vi "模拟控件转String.vi"(1 "Input":T2={"Digital Start Trigger Source 4"="/Dev1/PFI0", "Digital Start Trigger Edge 4"=10280, "min volt (V)"=0.0, "max volt (V)"=1.0, "rate"=100000.0, "device name"="Dev1", "Formula In"=[], "Total time (s)"=0.0} {"rate" format="%0.2f"; "max volt (V)" format="%0.2f"; "min volt (V)" format="%0.2f"; "Digital Start Trigger Edge 4" items=["Rising"=10280, "Falling"=10171]}) -> (0 "output":T1={"Digital Start Trigger Source 4"="/Dev1/PFI0", "Digital Start Trigger Edge 4"="", "minimum value"=-10.0, "maximum value"=10.0, "rate"=1000.0, "device name"="PXI1Slot5", "Total time"=0.0, "Formula In"=[]} {"rate" format="%0.2f"; "maximum value" format="%0.2f"; "minimum value" format="%0.2f"})   [LabVIEW 2021]
panel:
  # "1、formular in 中sample为各个分段函数的持续时间。\n2、Total time 为总时间，必须大于sample加起来的值。\n3、minimum value和maximum value默认±10V不改。\n4、rate为采样率，即时钟频率\n5、device name为选择的板卡名字，可选为PXI1Slot5-7\n6、Source 为接受触发的端口，Edge为选择上升沿触发\n还是其他类型触发。"
  # "In0：780 VCO 幅值（初始 0.6）\nIn1：780 VCO 频率（初始 0.7）"
  # "1、Formula In 中 sample 为各个函数的持续时间\n2、Total time 为总时间，必须大于 sample 之和\n3、min volt 和 max volt 默认±10V\n4、rate 为采样率，即时钟频率\n5、device name 为选择的板卡，可选为 Dev1\n6、Source 为接受触发的端口，Edge 为触发类型"
  # "In0：780 VCO 幅值（初始 0.6）\nIn1：780 VCO 频率（初始 0.7）"
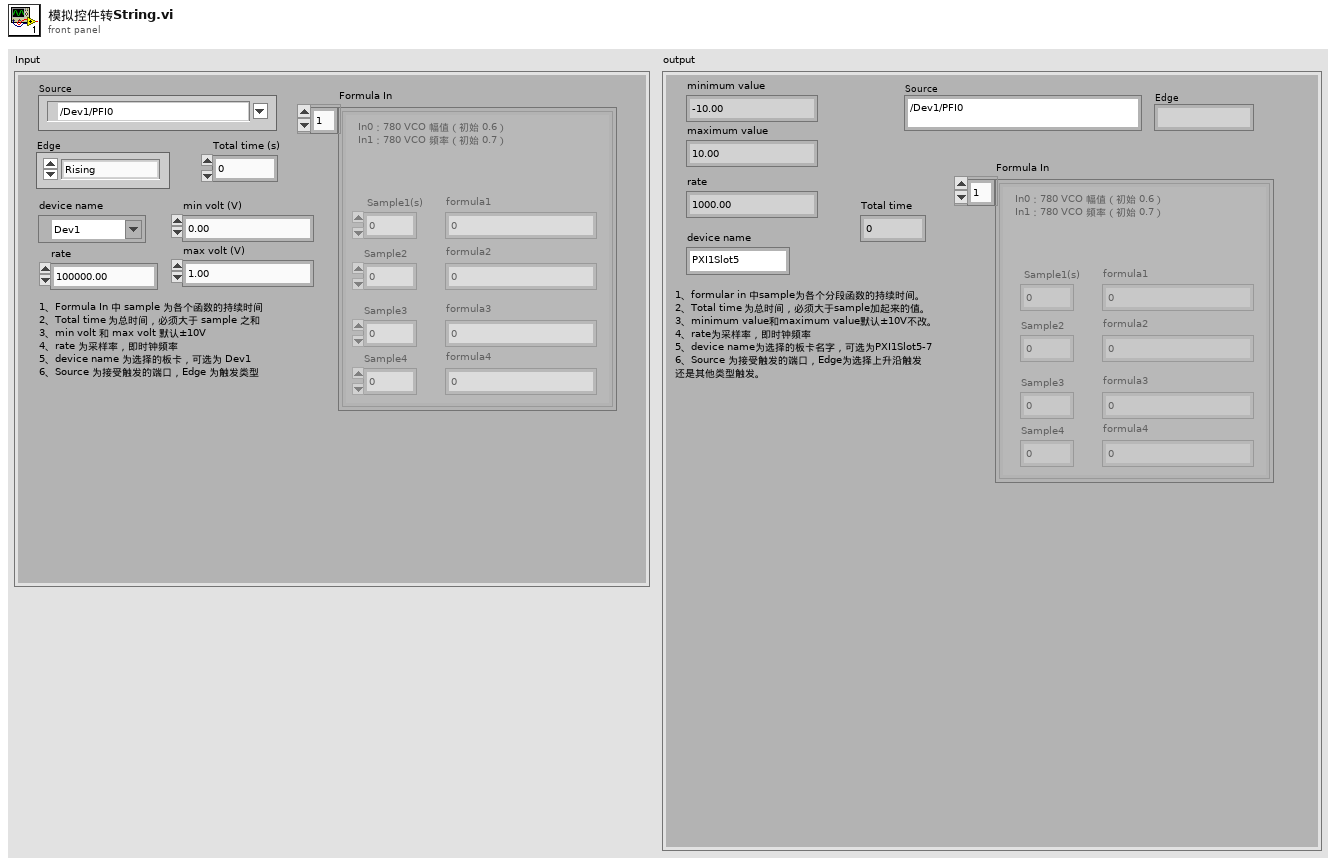
[diagram p1: front panel]
types:
  T1 = cluster{"Digital Start Trigger Source 4":string, "Digital Start Trigger Edge 4":string, "minimum value":dbl, "maximum value":dbl, "rate":dbl, "device name":string, "Total time":dbl, "Formula In":cluster{" Sample1(s)":dbl, "formula1":string, "Sample2":dbl, "formula2":string, "Sample3":dbl, "formula3":string, "Sample4":dbl, "formula4":string}[]}
  T2 = cluster{"Digital Start Trigger Source 4":tag, "Digital Start Trigger Edge 4":i32, "min volt (V)":dbl, "max volt (V)":dbl, "rate":dbl, "device name":tag, "Formula In":cluster{" Sample1(s)":dbl, "formula1":string, "Sample2":dbl, "formula2":string, "Sample3":dbl, "formula3":string, "Sample4":dbl, "formula4":string}[], "Total time (s)":dbl}
  T3 = cluster{" Sample1(s)":dbl, "formula1":string, "Sample2":dbl, "formula2":string, "Sample3":dbl, "formula3":string, "Sample4":dbl, "formula4":string}[]
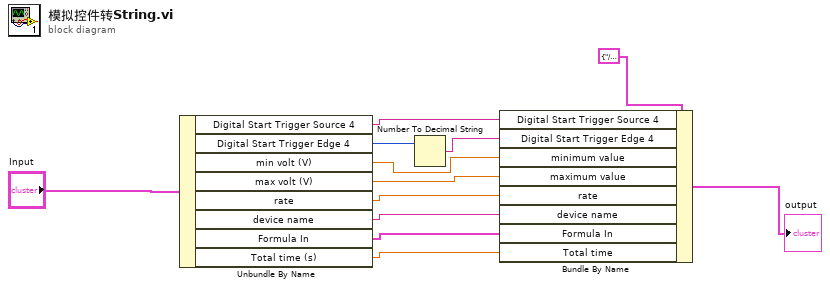
[diagram p0: block diagram]
diagram:
  n1 = Unbundle By Name("Input") -> ("Digital Start Trigger Source 4"=w9:tag, "Digital Start Trigger Edge 4"=w11:i32, "min volt (V)"=w7:dbl, "max volt (V)"=w6:dbl, "rate"=w5:dbl, "device name"=w4:tag, "Formula In"=w3:T3, "Total time (s)"=w2:dbl)
  n2 = Number To Decimal String(number=w11) -> (decimal integer string=w8:string)  [unwired: 1 in]
  n3 = Bundle By Name(cluster=T1 {"Digital Start Trigger Source 4"="/Dev1/PFI0", "Digital Start Trigger Edge 4"="", "minimum value"=-10.0, "maximum value"=10.0, "rate"=1000.0, "device name"="PXI1Slot5", "Total time"=0.0, "Formula In"=[{" Sample1(s)"=6.0, "formula1"="0.6", "Sample2"=0.0, "formula2"="0", "Sample3"=0.0, "formula3"="0", "Sample4"=0.0, "formula4"="0"}, {" Sample1(s)"=6.0, "formula1"="0.6", "Sample2"=0.0, "formula2"="0", "Sample3"=0.0, "formula3"="0", "Sample4"=0.0, "formula4"="0"}, {" Sample1(s)"=0.0, "formula1"="", "Sample2"=0.0, "formula2"="", "Sample3"=0.0, "formula3"="", "Sample4"=0.0, "formula4"=""}, {" Sample1(s)"=0.0, "formula1"="", "Sample2"=0.0, "formula2"="", "Sample3"=0.0, "formula3"="", "Sample4"=0.0, "formula4"=""}, {" Sample1(s)"=0.0, "formula1"="", "Sample2"=0.0, "formula2"="", "Sample3"=0.0, "formula3"="", "Sample4"=0.0, "formula4"=""}, {" Sample1(s)"=0.0, "formula1"="", "Sample2"=0.0, "formula2"="", "Sample3"=0.0, "formula3"="", "Sample4"=0.0, "formula4"=""}, {" Sample1(s)"=0.0, "formula1"="", "Sample2"=0.0, "formula2"="", "Sample3"=0.0, "formula3"="", "Sample4"=0.0, "formula4"=""}, {" Sample1(s)"=0.0, "formula1"="", "Sample2"=0.0, "formula2"="", "Sample3"=0.0, "formula3"="", "Sample4"=0.0, "formula4"=""}]} ("output"), "Digital Start Trigger Source 4"=w9, "Digital Start Trigger Edge 4"=w8, "minimum value"=w7, "maximum value"=w6, "rate"=w5, "device name"=w4, "Formula In"=w3, "Total time"=w2) -> (→"output":T1)
